vi "WPI_SerialPortRefNum Registry Get.vi"(8 "error in (no error)":errorcluster, 10 "refnum name":string="My Serial RefNum") -> (0 "error out":errorcluster, 3 "SerialPortRef":T1)   [LabVIEW 2017]
doc: "Gets the reference you specify. You first must set the reference with the RefNum Registry Set VI."
uses:
  <vilib>/Rock Robotics/WPI/SerialPort/WPI_SerialPortRef.ctl
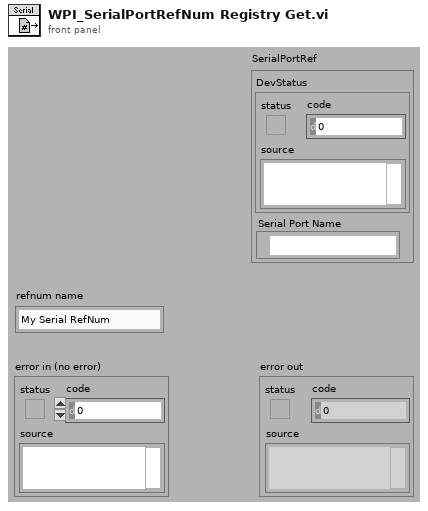
[diagram p1: front panel]
types:
  T1 = typedef "WPI_SerialPortRef.ctl" = cluster{"DevStatus":errorcluster, "Serial Port Name":refnum<visa-resource-name>}
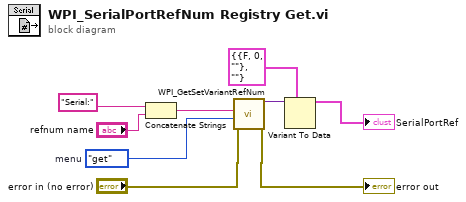
[diagram p0: block diagram]
diagram:
  w2 = enum16{"set", "get", "delete"}."get"  # menu
  n1 = Concatenate Strings("Serial:", "refnum name") -> (w9:string)
  n2 = call <vilib>:"WPI_GetSetVariantRefNum.vi"("error in (no error)"="error in (no error)", "Operation"=w2, "refnum name"=w9) -> ("error out"=→"error out":errorcluster, "DevRef"=w7:variant)  [unwired: 6 in, 1 out]
  n3 = Variant To Data(type=T1 {"DevStatus"={"status"=FALSE, "code"=0, "source"=""}, "Serial Port Name"=""} ("SerialPortRef"), Variant=w7) -> (data=→"SerialPortRef":T1)  [unwired: 1 in, 1 out]
